vi "Version 1_Read Decimal Places.vi"(7 "Unit ID (A)":string="A", 8 "error in":errorcluster, 10 "Software version (optional - wire for speed)":u8, 11 "VISA Session In":refnum<visa-resource-name>="Alicat") -> (0 "error out":errorcluster, 1 "Mass":i32, 2 "Volume":i32, 3 "VISA Session Out":refnum<visa-resource-name>, 4 "Pressure":i32)   [LabVIEW 2019]
doc: "Reads the decimal places of the pressure and flow rate variables."
uses:
  <vilib>/Instr/_visa.llb/VISA Flush IO Buffer Mask.ctl
panel:
  # "SW Version defaults to 0. \nIf un-wired, it will call a \nsub-VI to check."
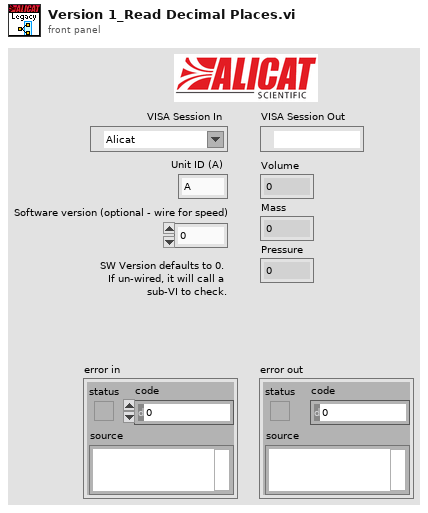
[diagram p1: front panel]
types:
  T1 = cluster{"Volume":i32, "AbsolutePressure":i32, "Mass":i32, "Gauge/Diff. Pressure":i32, "BarometricPressure":i32}
  T2 = typedef "VISA Flush IO Buffer Mask.ctl" = u16
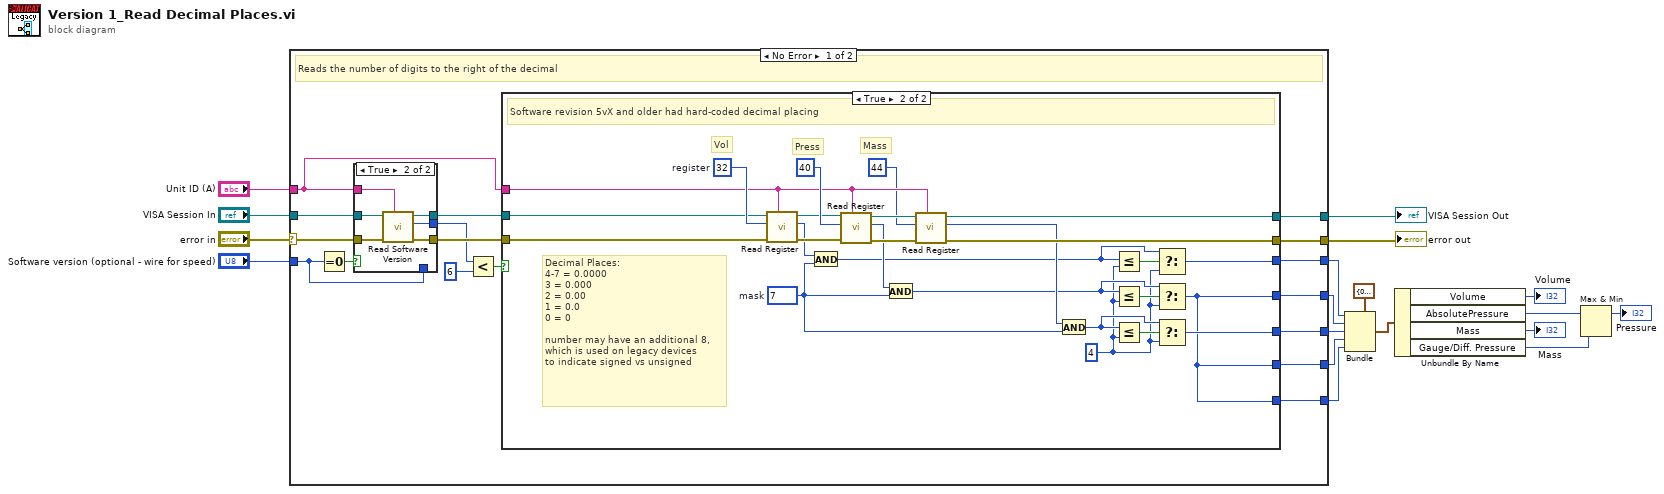
[diagram p0: block diagram]
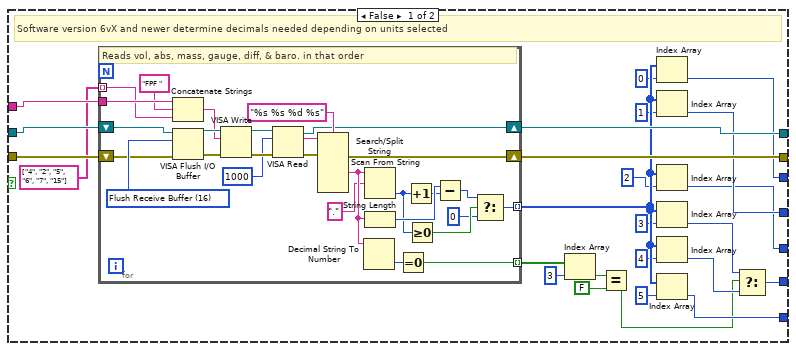
[diagram p3: hidden frame]
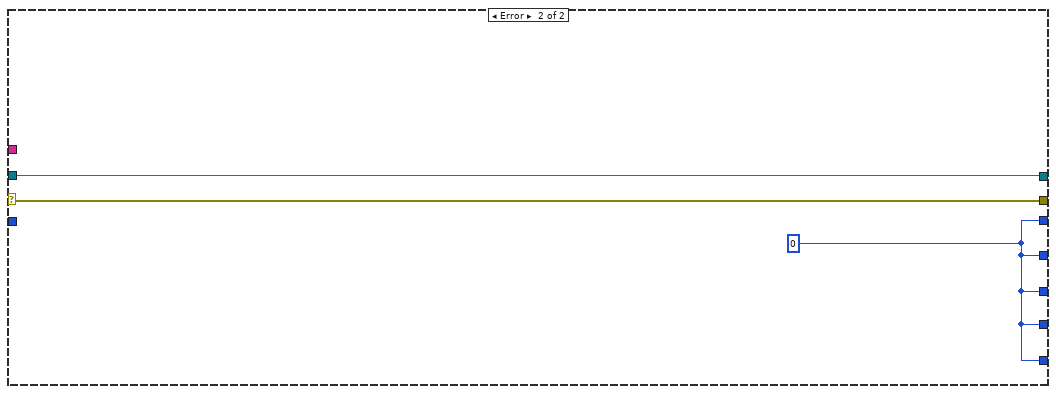
[diagram p4: hidden frame]
diagram:
  n1 = case shown="No Error" "error in" {
    selector: "error in" -> [w30 w125]
    tunnel: "VISA Session In" -> [w29 w126]
    tunnel: "Unit ID (A)" -> [w28 _]
    tunnel: [w35 w126] -> w16
    tunnel: [w34 w125] -> w15
    tunnel: [w33 w124] -> w11
    tunnel: [w32 w124] -> w10
    tunnel: [w31 w124] -> w9
    tunnel: [w22 w124] -> w8
    tunnel: [w21 w124] -> w7
    tunnel: "Software version (optional - wire for speed)" -> [w19 _]
    frame No Error {
      # "Reads the number of digits to the right of the decimal"
      n2 = Equal To 0?(x=w19) -> (x = 0?=w20:bool)
      n3 = case shown="True" w20 {
        tunnel: w30 -> [w37 w44]
        tunnel: w29 -> [w36 w43]
        tunnel: w28 -> [_ w42]
        tunnel: [w37 w41] -> w27
        tunnel: [w36 w40] -> w26
        tunnel: [w38 w39] -> w25
        tunnel: w19 -> [w38 _]
        frame False {
        }
        frame True {
          n4 = call "Read Software Version.vi"("Unit ID (A)"=w42, "error in"=w44, "VISA Session In"=w43) -> ("error out"=w41:errorcluster, "Software Version"=w39:u8, "VISA Session Out"=w40:refnum<visa-resource-name>)  [unwired: 6 in]
        }
      }
      n5 = Less?(x=w25, y=u8 6) -> (x < y?=w24:bool)
      n6 = case shown="True" w24 {
        tunnel: w26 -> [w68 w122]
        tunnel: w28 -> [w67 w119]
        tunnel: [w65 w115] -> w35
        tunnel: [w66 w114] -> w34
        tunnel: w27 -> [w69 w108]
        tunnel: [w55 w107] -> w33
        tunnel: [w54 w98] -> w32
        tunnel: [w53 w103] -> w31
        tunnel: [w59 w98] -> w22
        tunnel: [w56 w98] -> w21
        frame False {
          # "Software version 6vX and newer determine decimals needed depending on units selected"
          n7 = for {
            tunnel: w67 -> [w87]
            shift-right: [w84] -> w66
            shift-left: w69 -> [w93]
            shift-right: [w83] -> w65
            shift-left: w68 -> [w92]
            tunnel: string[] ["4", "2", "5", "6", "7", "15"] ("appended array") -> [w81] mode=indexing
            tunnel: [w73] -> w52 mode=indexing
            tunnel: [w78] -> w63 mode=indexing
            w96 = T2 16 items=["Flush Receive Buffer"=16, "Write Transmit Buffer to Device"=32, "Flush Receive Buffer (No I/O)"=64, "Flush Transmit Buffer"=128] ("Mask")
            # "Reads vol, abs, mass, gauge, diff, & baro. in that order"
            n8 = Concatenate Strings(w87, "FPF " ("format string (polled)"), w81) -> (w82:string)
            n9 = VISA Flush I/O Buffer(VISA resource name=w92, mask (16)=w96, error in (no error)=w93) -> (VISA resource name out=w89:refnum<visa-resource-name>, error out=w88:errorcluster)
            n10 = VISA Write(VISA resource name=w89, write buffer=w82, error in (no error)=w88) -> (VISA resource name out=w95:refnum<visa-resource-name>, error out=w97:errorcluster)  [unwired: 1 out]
            n11 = VISA Read(VISA resource name=w95, byte count=u32 1000, error in (no error)=w97) -> (VISA resource name out=w83:refnum<visa-resource-name>, read buffer=w90:string, error out=w85:errorcluster)  [unwired: 1 out]
            n12 = Scan From String(format string="%s %s %d %s", input string=w90, error in=w85) -> (error out=w84:errorcluster, output 2=w77:string)  [unwired: 8 in, 2 out]
            n13 = Decimal String To Number(string=w77) -> (number=w79:i32)  [unwired: 2 in, 1 out]
            n14 = Search/Split String(string=w77, search string/char (-)="." ("regular expression")) -> (offset of match=w74:i32)  [unwired: 1 in, 2 out]
            n15 = String Length(string=w77) -> (length=w80:i32)
            n16 = Equal To 0?(x=w79) -> (x = 0?=w78:bool)
            n17 = Increment(x=w74) -> (x+1=w75:i32)
            n18 = Greater Or Equal To 0?(x=w74) -> (x >= 0?=w71:bool)
            n19 = Subtract(x=w80, y=w75) -> (x-y=w72:i32)
            n20 = Select(t=w72, s=w71, f=0) -> (s? t:f=w73:i32)
          }
          n21 = Index Array(array=w63, index=3) -> (element=w61:bool)
          n22 = Equal?(x=w61, y=FALSE) -> (x = y?=w45:bool)
          n23 = Index Array(array=w52, index=0) -> (element=w55:i32)
          n24 = Index Array(array=w52, index=1) -> (element=w54:i32)
          n25 = Index Array(array=w52, index=2) -> (element=w53:i32)
          n26 = Index Array(array=w52, index=3) -> (element=w58:i32)
          n27 = Index Array(array=w52, index=4) -> (element=w57:i32)
          n28 = Index Array(array=w52, index=5) -> (element=w56:i32)
          n29 = Select(t=w58, s=w45, f=w57) -> (s? t:f=w59:i32)
        }
        frame True {
          w99 = 4 ("y")
          w109 = 7  # mask
          w123 = u16 32  # register
          # "Decimal Places:\n4-7 = 0.0000\n3 = 0.000\n2 = 0.00\n1 = 0.0\n0 = 0\n\nnumber may have an additional 8,\nwhich is used on legacy devices \nto indicate signed vs unsigned"
          # "Mass"
          # "Press"
          # "Vol"
          # "Software revision 5vX and older had hard-coded decimal placing"
          n30 = call "Read Register.vi"("Unit ID (A)"=w119, "error in"=w108, "Register address"=w123, "VISA Session In"=w122) -> ("error out"=w118:errorcluster, "Register Value (I32)"=w112:i32, "VISA Session Out"=w120:refnum<visa-resource-name>)  [unwired: 5 in]
          n31 = And(x=w112, y=w109) -> (x .and. y?=w100:i32)
          n32 = call "Read Register.vi"("Unit ID (A)"=w119, "error in"=w118, "Register address"=u16 40, "VISA Session In"=w120) -> ("error out"=w117:errorcluster, "Register Value (I32)"=w110:i32, "VISA Session Out"=w116:refnum<visa-resource-name>)  [unwired: 5 in]
          n33 = And(x=w110, y=w109) -> (x .and. y?=w101:i32)
          n34 = call "Read Register.vi"("Unit ID (A)"=w119, "error in"=w117, "Register address"=u16 44, "VISA Session In"=w116) -> ("error out"=w114:errorcluster, "Register Value (I32)"=w111:i32, "VISA Session Out"=w115:refnum<visa-resource-name>)  [unwired: 5 in]
          n35 = And(x=w111, y=w109) -> (x .and. y?=w102:i32)
          n36 = Less Or Equal?(x=w100, y=w99) -> (x <= y?=w106:bool)
          n37 = Less Or Equal?(x=w101, y=w99) -> (x <= y?=w105:bool)
          n38 = Less Or Equal?(x=w102, y=w99) -> (x <= y?=w104:bool)
          n39 = Select(t=w100, s=w106, f=w99) -> (s? t:f=w107:i32)
          n40 = Select(t=w101, s=w105, f=w99) -> (s? t:f=w98:i32)
          n41 = Select(t=w102, s=w104, f=w99) -> (s? t:f=w103:i32)
        }
      }
    }
    frame Error {
      w124 = 0
    }
  }
  "error out" <- w15
  "VISA Session Out" <- w16
  n42 = Bundle(cluster=T1 {"Volume"=0, "AbsolutePressure"=0, "Mass"=0, "Gauge/Diff. Pressure"=0, "BarometricPressure"=0} ("output cluster"), "Volume"=w11, "AbsolutePressure"=w10, "Mass"=w9, "Gauge/Diff. Pressure"=w8, "BarometricPressure"=w7) -> (w6:T1)
  n43 = Unbundle By Name(w6) -> ("Volume"=→"Volume":i32, "AbsolutePressure"=w5:i32, "Mass"=→"Mass":i32, "Gauge/Diff. Pressure"=w4:i32)
  n44 = Max & Min(x=w5, y=w4) -> (max(x,y)=→"Pressure":i32)  [unwired: 1 out]
